vi "U8Array-toU32Array_128bit.vi"(11 "16 x U8":u8[](array[numeric]) format="%.0x") -> (3 "4 x U32":u32[](array[numeric]) format="%.0x")   [LabVIEW 2017]
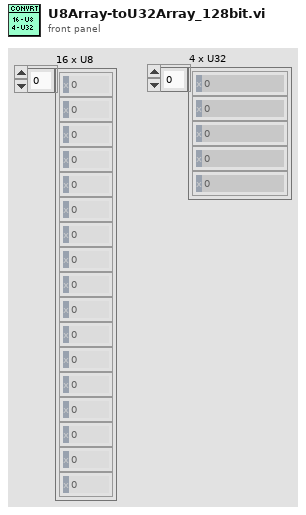
[diagram p1: front panel]
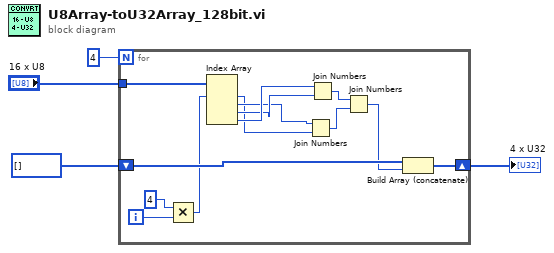
[diagram p0: block diagram]
diagram:
  n1 = for {
    N: 4 -> [_]
    shift-right: [w12] -> w4
    shift-left: u32[] [] -> [w17]
    tunnel: "16 x U8" -> [w16]
    i -> [w15]
    n2 = Multiply(x=4, y=w15) -> (x*y=w13:i32)
    n3 = Index Array(array=w16, index #1=w13) -> (element #1=w5:u8, element #2=w6:u8, element #3=w7:u8, element #4=w8:u8)  [unwired: 3 in]
    n4 = Join Numbers(hi=w6, lo=w5) -> ((hi.lo)=w9:u16)
    n5 = Join Numbers(hi=w8, lo=w7) -> ((hi.lo)=w11:u16)
    n6 = Join Numbers(hi=w11, lo=w9) -> ((hi.lo)=w10:u32)
    n7 = Build Array (concatenate)(w17, w10) -> (w12:u32[])
  }
  "4 x U32" <- w4
